vi "SQL_monitor_data_settinngs_update.vi"(8 "报警信息设置":string[][](table), 11 "工作条件及报警门限参考值设定":string[][](table)) -> (3 "error out":errorcluster)   [LabVIEW 2014]
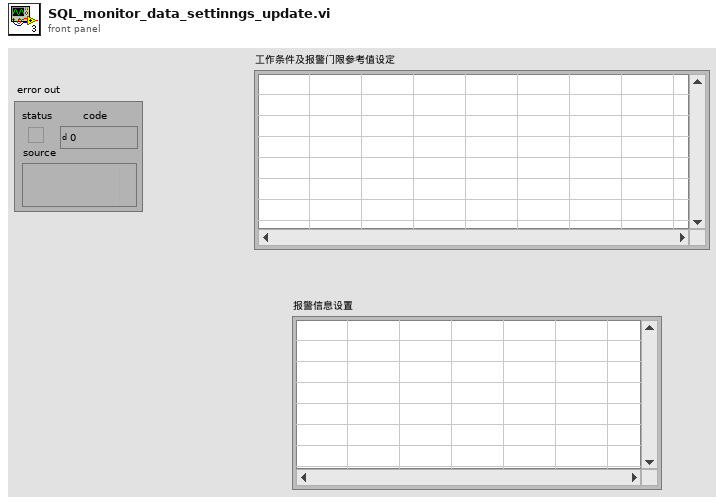
[diagram p1: front panel]
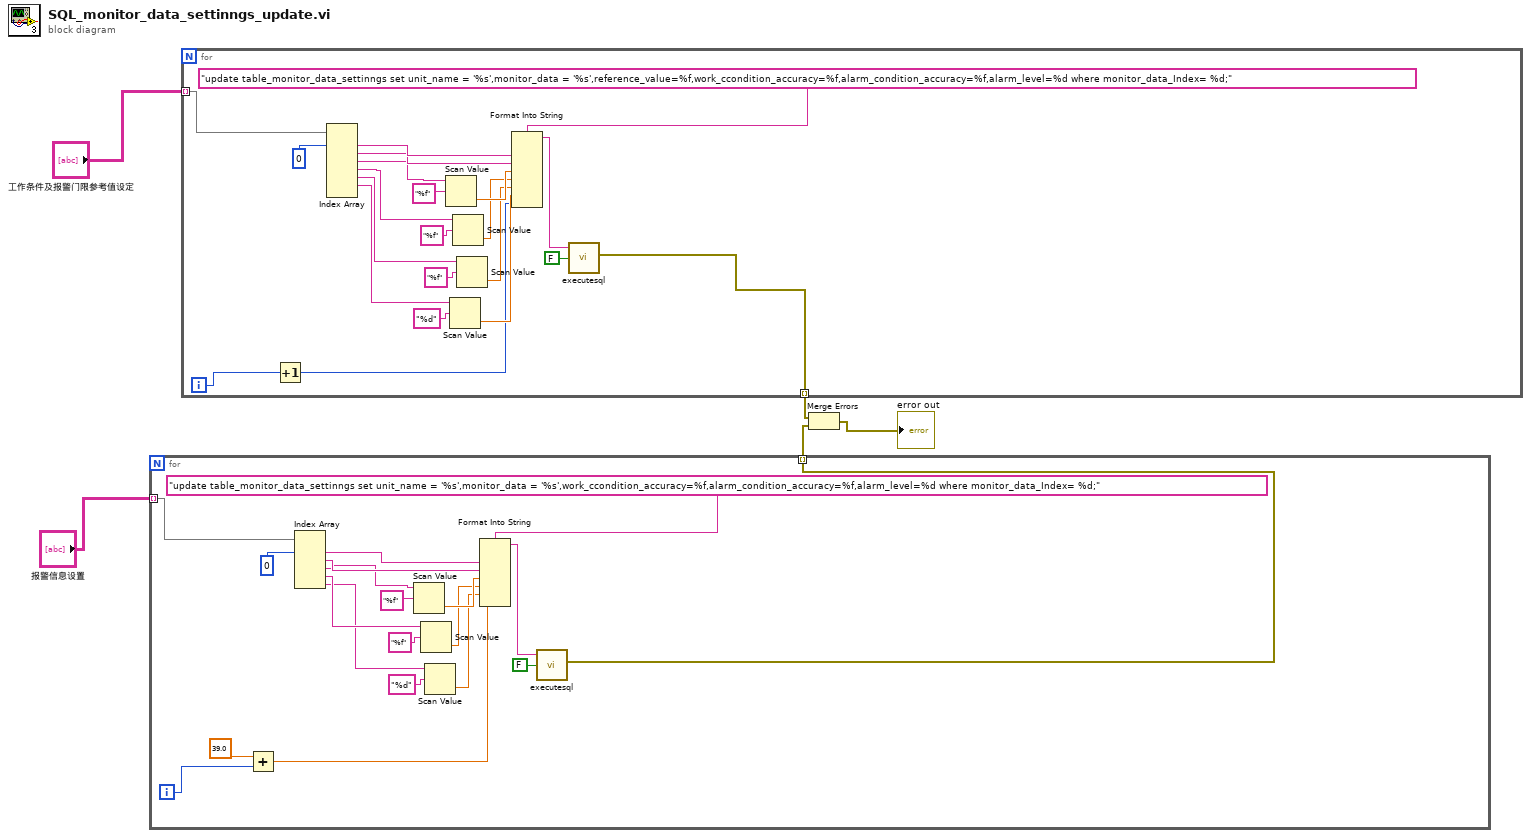
[diagram p0: block diagram]
diagram:
  n1 = for {
    tunnel: "报警信息设置" -> [w21] mode=indexing
    tunnel: [w6] -> w2 mode=indexing
    i -> [w7]
    n2 = Add(x=39.0, y=w7) -> (x+y=w9:dbl)
    n3 = Index Array(array=w21, index #1=0 ("索引")) -> (element #1=w14:string, element #2=w13:string, element #3=w12:string, element #4=w11:string, element #5=w10:string)  [unwired: 4 in]
    n4 = Scan Value(string=w12, format string="%f" ("格式字符串")) -> (value=w18:dbl)  [unwired: 1 in, 1 out]
    n5 = Scan Value(string=w11, format string="%f" ("格式字符串")) -> (value=w17:dbl)  [unwired: 1 in, 1 out]
    n6 = Scan Value(string=w10, format string="%d" ("格式字符串")) -> (value=w15:dbl)  [unwired: 1 in, 1 out]
    n7 = Format Into String(format string="update table_monitor_data_settinngs set unit_name = '%s',monitor_data = '%s',work_ccondition_accuracy=%f,alarm_condition_accuracy=%f,alarm_level=%d where monitor_data_Index= %d;", w14, w13, w18, w17, w15, w9) -> (resulting string=w23:string)  [unwired: 2 in, 1 out]
    n8 = call "executesql.vi"("Return Data (T)"=FALSE, "Command Text"=w23) -> ("error out"=w6:errorcluster)  [unwired: 5 in, 1 out]
  }
  n9 = for {
    tunnel: "工作条件及报警门限参考值设定" -> [w42] mode=indexing
    tunnel: [w26] -> w3 mode=indexing
    i -> [w39]
    n10 = Increment(x=w39) -> (x+1=w27:i32)
    n11 = Index Array(array=w42, index #1=0 ("索引")) -> (element #1=w45:string, element #2=w38:string, element #3=w37:string, element #4=w34:string, element #5=w31:string, element #6=w29:string)  [unwired: 6 in, 1 out]
    n12 = Scan Value(string=w37, format string="%f" ("格式字符串")) -> (value=w36:dbl)  [unwired: 1 in, 1 out]
    n13 = Scan Value(string=w29, format string="%d" ("格式字符串")) -> (value=w28:dbl)  [unwired: 1 in, 1 out]
    n14 = Scan Value(string=w34, format string="%f" ("格式字符串")) -> (value=w35:dbl)  [unwired: 1 in, 1 out]
    n15 = Scan Value(string=w31, format string="%f" ("格式字符串")) -> (value=w30:dbl)  [unwired: 1 in, 1 out]
    n16 = Format Into String(format string="update table_monitor_data_settinngs set unit_name = '%s',monitor_data = '%s',reference_value=%f,work_ccondition_accuracy=%f,alarm_condition_accuracy=%f,alarm_level=%d where monitor_data_Index= %d;", w45, w38, w36, w35, w30, w28, w27) -> (resulting string=w44:string)  [unwired: 2 in, 1 out]
    n17 = call "executesql.vi"("Return Data (T)"=FALSE, "Command Text"=w44) -> ("error out"=w26:errorcluster)  [unwired: 5 in, 1 out]
  }
  n18 = Merge Errors(w3, w2) -> (→"error out":errorcluster)
